vi "json Insert I64 Array - string path.vi"(8 "error in (no error)":errorcluster, 9 "anything":i64[](array[numeric]), 10 "path":string, 11 "JSON Document in":refnum<class "JSON Document.lvclass">) -> (0 "error out":errorcluster, 1 "replaced?":bool, 3 "JSON Document out":refnum<class "JSON Document.lvclass">)   [LabVIEW 2016, in "JSON Document.lvclass"]
uses:
  JSON Document.lvclass
  JSON Document.lvclass/JSON Document.ctl
  json Insert - String Path.vi
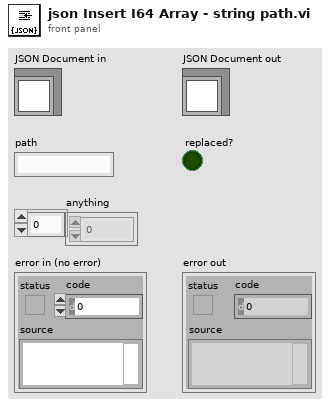
[diagram p1: front panel]
types:
  T1 = cluster{"enable extensions?":bool, "allow comments?":bool}
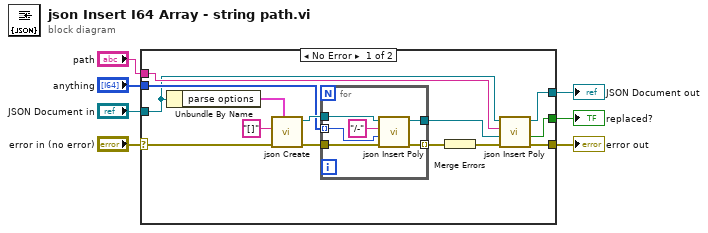
[diagram p0: block diagram]
diagram:
  n1 = case shown="No Error" "error in (no error)" {
    selector: "error in (no error)" -> [w10 w29]
    tunnel: [w21 w29] -> w6
    tunnel: [w14 w28] -> w4
    tunnel: "JSON Document in" -> [w9 w28]
    tunnel: "anything" -> [w17 _]
    tunnel: "path" -> [w11 _]
    tunnel: [w20 _] -> w1
    frame No Error {
      n2 = Unbundle By Name(w9) -> ("parse options"=w8:T1)
      n3 = call "json Create.vi"("options"=w8, "error in (no error)"=w10, "JSON String"="[]") -> ("error out"=w13:errorcluster, "JSON Document out"=w18:refnum<class "JSON Document.lvclass">)  [unwired: 7 in]
      n4 = for {
        tunnel: w18 -> [w27]
        tunnel: w17 -> [w26] mode=indexing
        tunnel: w13 -> [w25]
        tunnel: [w24] -> w16 mode=indexing
        tunnel: [w23] -> w12
        n5 = call-poly "json Insert Poly.vi"("error in (no error)"=w25, "anything"=w26, "path"="/-" ("initial string"), "JSON Document in"=w27) -> ("error out"=w24:errorcluster, "JSON Document out"=w23:refnum<class "JSON Document.lvclass">)  [unwired: 5 in, 1 out]
      }
      n6 = Merge Errors(w16) -> (w15:errorcluster)
      n7 = call-poly "json Insert Poly.vi"("error in (no error)"=w15, "anything"=w12, "path"=w11, "JSON Document in"=w9) -> ("error out"=w21:errorcluster, "replaced?"=w20:bool, "JSON Document out"=w14:refnum<class "JSON Document.lvclass">)  [unwired: 5 in]
    }
    frame Error {
    }
  }
  "error out" <- w6
  "JSON Document out" <- w4
  "replaced?" <- w1
